vi "Sleep.vi"(8 "error in (no error)":errorcluster caption="错误输入（无错误）", 10 "等待时间（毫秒）":u32) -> (0 "error out":errorcluster caption="错误输出")   [LabVIEW 2018]
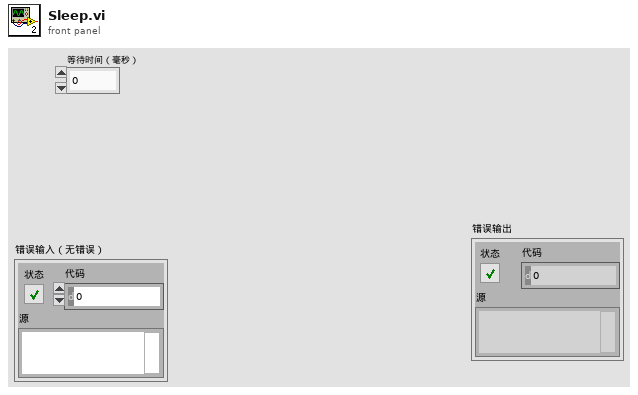
[diagram p1: front panel]
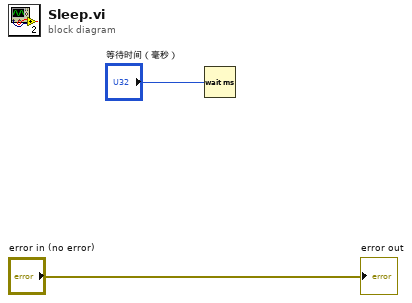
[diagram p0: block diagram]
diagram:
  n1 = Wait (ms)(milliseconds to wait="等待时间（毫秒）") -> ()  [unwired: 1 out]
  "error out" <- "error in (no error)"
